vi "Start Polling.vi"(8 "Error In":errorcluster, 11 "CS++BaseActor in":refnum<class "CS++BaseActor.lvclass">) -> (0 "Error Out":errorcluster, 3 "CS++BaseActor out":refnum<class "CS++BaseActor.lvclass">)   [LabVIEW 2015, in "CS++BaseActor.lvlib" / "CS++BaseActor.lvclass"]
doc: "Start polling if polling intervall is less equal 0s."
uses:
  CS++BaseActor.lvclass
  CS++BaseActor.lvclass/CS++BaseActor.ctl
  Classes/CS++ProcessVariables/ProcessVariable/PV.lvclass
  Classes/CS++ProcessVariables/ProcessVariable/PV.lvclass/PV.ctl
  CS++BaseActor Messages/Polling Msg/Polling Msg.lvclass
  <vilib>/ActorFramework/Actor/Actor.lvclass/Actor.ctl
  <vilib>/ActorFramework/Message Enqueuer/Message Enqueuer.lvclass/Message Enqueuer.ctl
  Classes/CS++ProcessVariables/ProcessVariable/Write Timestamp.vi
  Classes/CS++ProcessVariables/ProcessVariable/Write Data.vi
  <vilib>/ActorFramework/Message Enqueuer/Init from Existing Queue.vi
  <vilib>/ActorFramework/Message Enqueuer/Message Enqueuer.lvclass
  <vilib>/ActorFramework/Actor/Actor.lvclass
  Classes/CS++ProcessVariables/PVConnection/PVConnection.lvclass
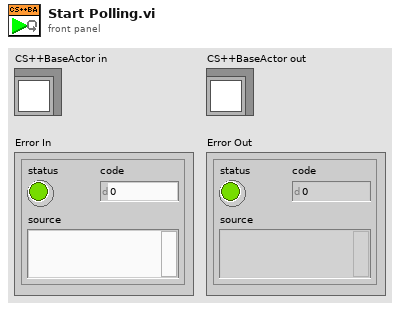
[diagram p1: front panel]
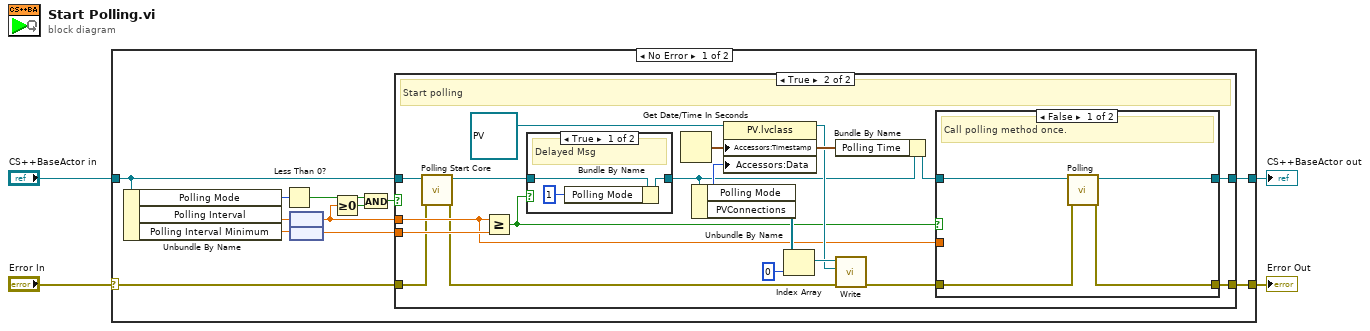
[diagram p0: block diagram]
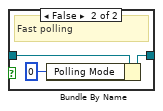
[diagram p3: hidden frame]
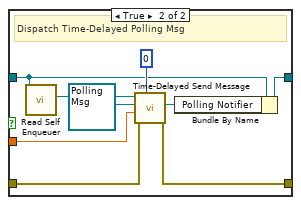
[diagram p4: hidden frame]
diagram:
  n1 = case shown="No Error" "Error In" {
    selector: "Error In" -> [w12 w58]
    tunnel: [w11 w58] -> w3
    tunnel: [w13 w57] -> w1
    tunnel: "CS++BaseActor in" -> [w14 w57]
    frame No Error {
      n2 = Unbundle By Name(w14) -> ("Polling Mode"=w16:i32, "Polling Interval"=w15:dbl[unit], "Polling Interval Minimum"=w6:dbl[unit])
      n3 = Less Than 0?(x=w16) -> (x < 0?=w10:bool)
      n4 = node(w15) -> (w7:dbl)
      n5 = node(w6) -> (w5:dbl)
      n6 = Greater Or Equal To 0?(x=w7) -> (x >= 0?=w8:bool)
      n7 = And(x=w10, y=w8) -> (x .and. y?=w9:bool)
      n8 = case shown="True" w9 {
        tunnel: w14 -> [w18 w22]
        tunnel: [w18 w34] -> w13
        tunnel: w12 -> [w17 w20]
        tunnel: [w17 w28] -> w11
        tunnel: w7 -> [_ w24]
        tunnel: w5 -> [_ w25]
        frame False {
          # "Don't start polling"
        }
        frame True {
          # "Start polling"
          n9 = call-dynamic "Polling Start Core.vi"("Error In"=w20, "CS++BaseActor in"=w22) -> ("Error Out"=w19:errorcluster, "CS++BaseActor out"=w21:refnum<class "CS++BaseActor.lvclass">)  [unwired: 8 in]
          n10 = Greater Or Equal?(x=w24, y=w25) -> (x >= y?=w23:bool)
          n11 = case shown="True" w23 {
            tunnel: w21 -> [w39 w42]
            tunnel: [w38 w41] -> w26
            frame True {
              # "Delayed Msg"
              n12 = Bundle By Name(cluster=w39, "Polling Mode"=1) -> (w38:refnum<class "CS++BaseActor.lvclass">)
            }
            frame False {
              # "Fast polling"
              n13 = Bundle By Name(cluster=w42, "Polling Mode"=0) -> (w41:refnum<class "CS++BaseActor.lvclass">)
            }
          }
          n14 = Get Date/Time In Seconds() -> (seconds since 1Jan1904=w32:timestamp)
          n15 = Unbundle By Name(w26) -> ("Polling Mode"=w31:i32, "PVConnections"=w35:refnum<class "PVConnection.lvclass">[])
          n16 = property class="PV.lvclass"(reference=refnum<class "PV.lvclass"> refnum ("CS++ProcessVariables.lvlib:PV.lvclass"), "Accessors:Timestamp"=w32, "Accessors:Data"=w31) -> (reference out=w29:refnum<class "PV.lvclass">)  [unwired: 1 in, 1 out]
          n17 = Index Array(array=w35, index=0) -> (element=w30:refnum<class "PVConnection.lvclass">)
          n18 = Bundle By Name(cluster=w26, "Polling Time"=w32) -> (w37:refnum<class "CS++BaseActor.lvclass">)
          n19 = call "Write.vi"("error in (no error)"=w19, "PV"=w29, "PVConnection in"=w30) -> ("error out"=w27:errorcluster)  [unwired: 7 in, 1 out]
          n20 = case shown="False" w23 {
            tunnel: w27 -> [w47 w55]
            tunnel: [w46 w54] -> w28
            tunnel: w37 -> [w44 w50]
            tunnel: [w45 w49] -> w34
            tunnel: w24 -> [_ w51]
            frame False {
              # "Call polling method once."
              n21 = call "Polling.vi"("Error In"=w47, "CS++BaseActor in"=w44) -> ("Error Out"=w46:errorcluster, "CS++BaseActor out"=w45:refnum<class "CS++BaseActor.lvclass">)  [unwired: 8 in]
            }
            frame True {
              # "Dispatch Time-Delayed Polling Msg"
              n22 = call <vilib>:"Read Self Enqueuer.vi"("Actor"=w50) -> ("Self Enqueuer"=w56:refnum<class "Message Enqueuer.lvclass">)  [unwired: 10 in]
              n23 = call <vilib>:"Time-Delayed Send Message.vi"("# Copies (0 = infinite repeat)"=u32 0, "error in (no error)"=w55, "Milliseconds To Wait"=w51, "Message"=refnum<class "Polling Msg.lvclass"> refnum ("CS++BaseActor.lvlib:Polling Msg.lvclass"), "Message Enqueuer"=w56) -> ("error out"=w54:errorcluster, "Delivery Notifier"=w48:refnum<notifier>)  [unwired: 5 in]
              n24 = Bundle By Name(cluster=w50, "Polling Notifier"=w48) -> (w49:refnum<class "CS++BaseActor.lvclass">)
            }
          }
        }
      }
    }
    frame Error {
    }
  }
  "Error Out" <- w3
  "CS++BaseActor out" <- w1
